vi "calc 3-phase ESR.vi"(7 "Acquisition mode":T1, 8 "error in":errorcluster, 10 "InverterWaveforms":T9, 11 "Processing loop variables":T2 {"CurrInverter"."last updated" format="%<%H:%M\n%d/%m/%Y>T"; "CurrInverter"."set flag" items=["False", "True"]}) -> (0 "error out":errorcluster, 1 "Max ESR":dbl[](array[numeric]), 2 "Raw ESR sum":dbl[](array[numeric]), 3 "Processing loop variables":T2 {"CurrInverter"."last updated" format="%<%H:%M\n%d/%m/%Y>T"; "CurrInverter"."set flag" items=["False", "True"]})   [LabVIEW 2019, in "Main.lvclass"]
doc: "Developed by Kevin Thompson\nkevin@thompsonengineering.net\n\nCopyright 2020\nThompson Engineering, LLC"
uses:
  Main.lvclass
  Common/DataTypes/InverterWaveforms--cluster.ctl
  Common/DataTypes/ChannelWaveforms--cluster.ctl
  DataTypes/Processing loop variables--cluster.ctl
  DataTypes/averaging variables.ctl
  DataTypes/ESR alarm variables.ctl
  Common/DataTypes/Inverter database record v2--cluster.ctl
  Common/DataTypes/inverter info v2--cluster.ctl
  Common/DataTypes/inverter gain range--cluster.ctl
  Common/DataTypes/inverter offset range--cluster.ctl
  Common/DataTypes/Acquisition Mode--cluster.ctl
  <vilib>/Analysis/baseanly.llb/Mean (DBL).vi
  <vilib>/Analysis/NI_AALPro.lvlib
  <vilib>/Analysis/NI_AALBase.lvlib
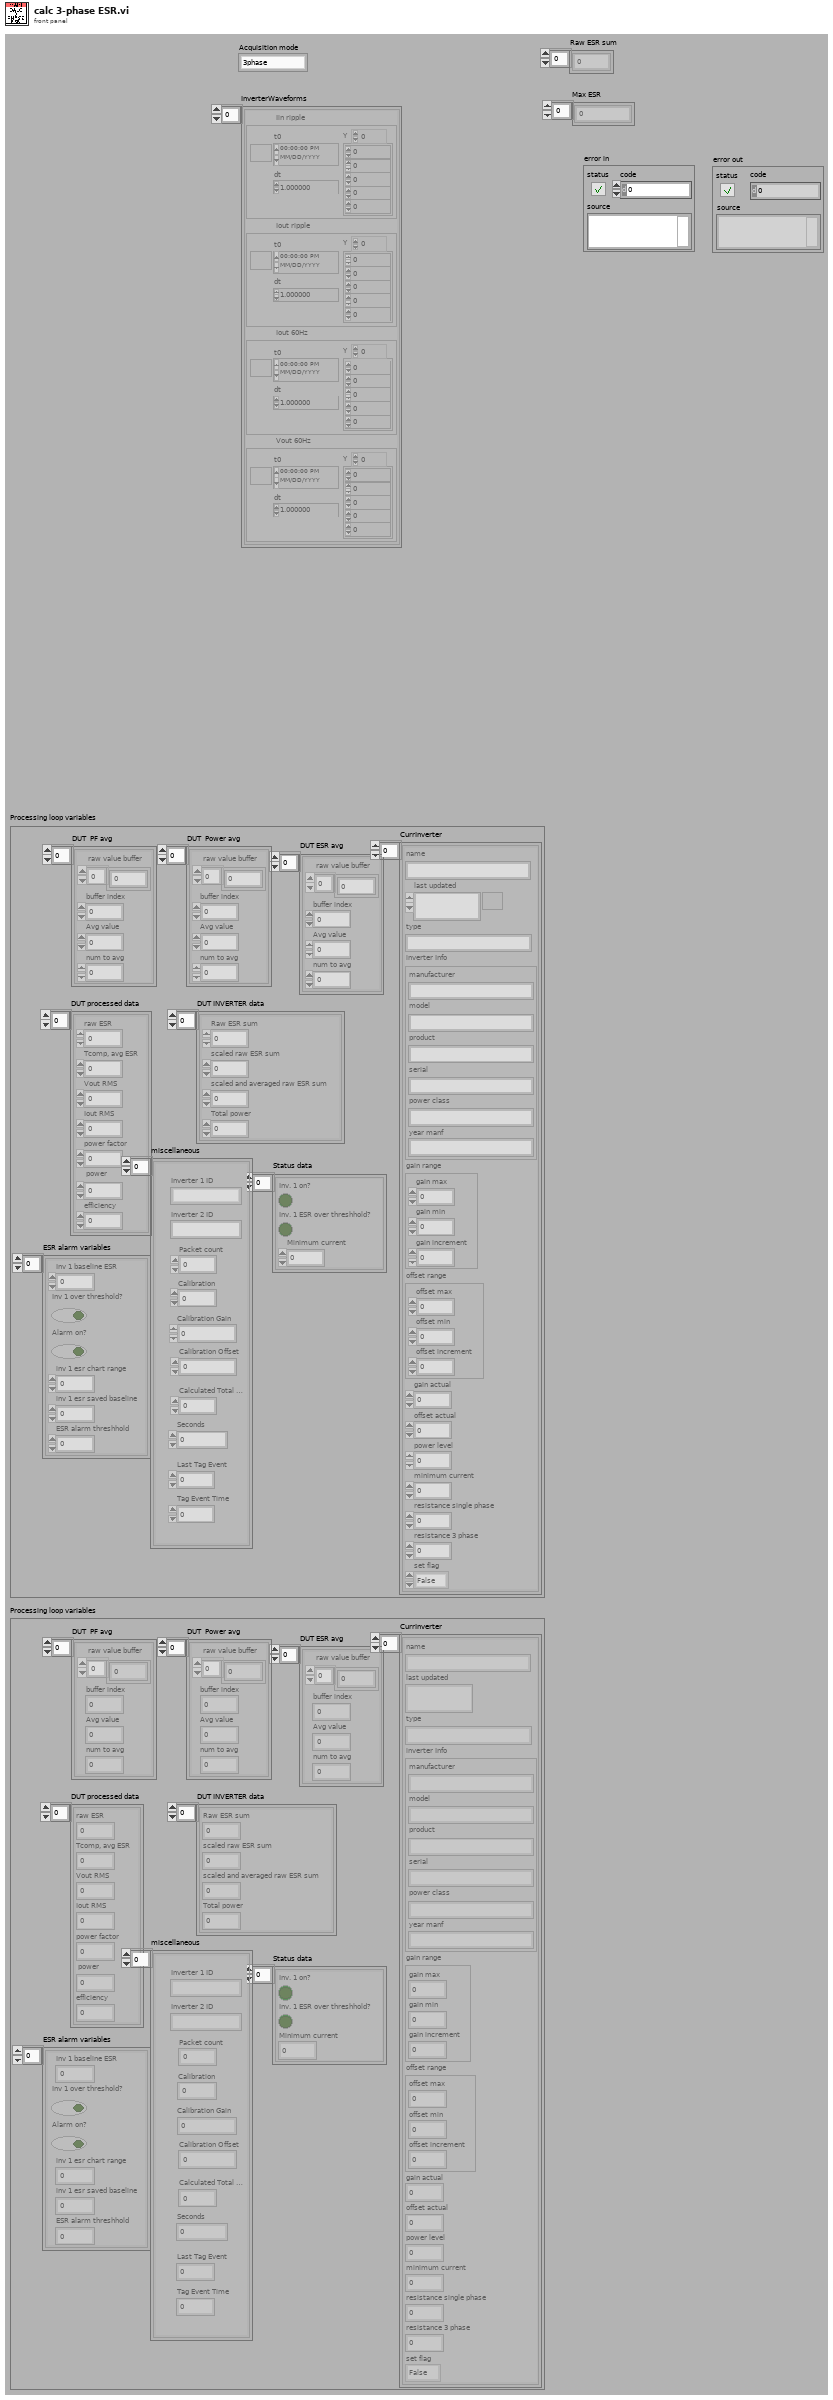
[diagram p1: front panel]
types:
  T1 = typedef "Acquisition Mode--cluster.ctl" = enum16{"3phase", "Single"}
  T2 = typedef "Main.lvclass/Processing loop variables--cluster.ctl" = cluster{"DUT ESR avg":T3[], "DUT  PF avg":T3[], "DUT  Power avg ":T3[], "DUT processed data":cluster{"raw ESR":dbl, "Tcomp, avg ESR":dbl, "Vout RMS":dbl, "Iout RMS":dbl, "power factor":dbl, "power":dbl, "efficiency":dbl}[], "ESR alarm variables":T4[], "Status data":cluster{"Inv. 1 on?":bool, "Inv. 1 ESR over threshhold?":bool, "Minimum current":dbl}[], "CurrInverter":T5[], "miscellaneous":cluster{"Inverter 1 ID":string, "Inverter 2 ID":string, "Packet count":u32, "Calibration":dbl, "Calibration Gain":dbl, "Calibration Offset":dbl, "Calculated Total Power":dbl, "Seconds":dbl, "Last Tag Event":dbl, "Tag Event Time":dbl}[], "DUT INVERTER data":cluster{"Raw ESR sum":dbl, "scaled raw ESR sum":dbl, "scaled and averaged raw ESR sum":dbl, "Total power":dbl}[]}
  T3 = typedef "Main.lvclass/averaging variables.ctl" = cluster{"raw value buffer":dbl[], "buffer index":i32, "Avg value":dbl, "num to avg":i32}
  T4 = typedef "Main.lvclass/ESR alarm variables.ctl" = cluster{"Inv 1 baseline ESR":dbl, "Inv 1 over threshold?":bool, "Alarm on?":bool, "inv 1 esr chart range":dbl, "inv 1 esr saved baseline":dbl, "ESR alarm threshhold":dbl}
  T5 = typedef "Inverter database record v2--cluster.ctl" = cluster{"name":string, "last updated":timestamp, "type":string, "inverter Info":T6, "gain range":T7, "offset range":T8, "gain actual":dbl, "offset actual":dbl, "power level":dbl, "minimum current":dbl, "resistance single phase":dbl, "resistance 3 phase":dbl, "set flag":u16}
  T6 = typedef "inverter info v2--cluster.ctl" = cluster{"manufacturer":string, "model":string, "product":string, "serial":string, "power class":string, "year manf":string}
  T7 = typedef "inverter gain range--cluster.ctl" = cluster{"gain max":dbl, "gain min":dbl, "gain increment":dbl}
  T8 = typedef "inverter offset range--cluster.ctl" = cluster{"offset max":dbl, "offset min":dbl, "offset increment":dbl}
  T9 = typedef "InverterWaveforms--cluster.ctl" = T10[]
  T10 = typedef "ChannelWaveforms--cluster.ctl" = cluster{"Iin ripple ":waveform(dbl), "Iout ripple ":waveform(dbl), "Iout 60Hz":waveform(dbl), "Vout 60Hz":waveform(dbl)}
  T11 = cluster{"raw ESR":dbl, "Tcomp, avg ESR":dbl, "Vout RMS":dbl, "Iout RMS":dbl, "power factor":dbl, "power":dbl, "efficiency":dbl}[]
  T12 = cluster{"Raw ESR sum":dbl, "scaled raw ESR sum":dbl, "scaled and averaged raw ESR sum":dbl, "Total power":dbl}[]
  T13 = cluster{"Raw ESR sum":dbl, "scaled raw ESR sum":dbl, "scaled and averaged raw ESR sum":dbl, "Total power":dbl}
  T14 = cluster{"raw ESR":dbl, "Tcomp, avg ESR":dbl, "Vout RMS":dbl, "Iout RMS":dbl, "power factor":dbl, "power":dbl, "efficiency":dbl}
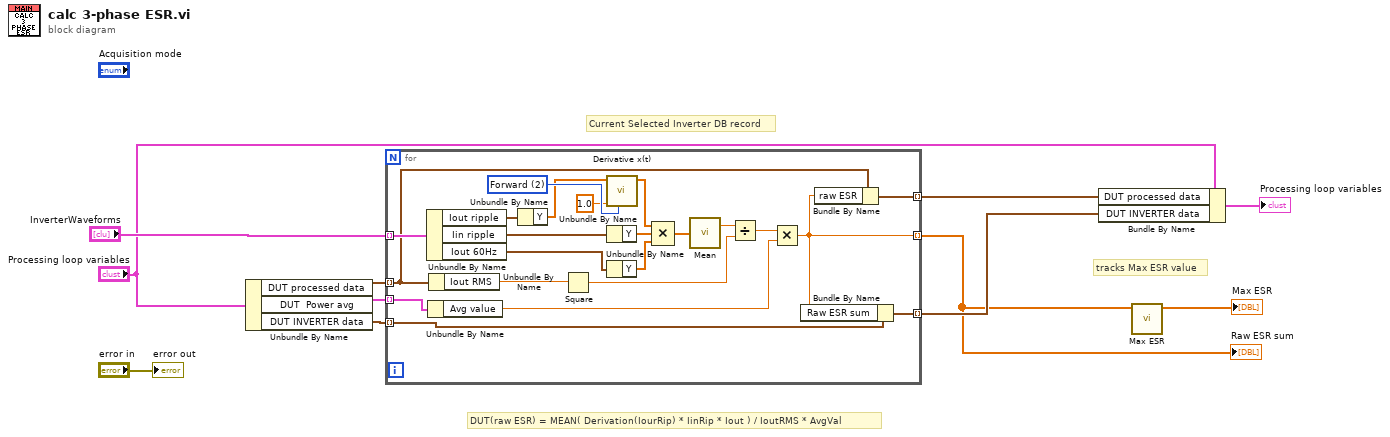
[diagram p0: block diagram]
diagram:
  # "DUT(raw ESR) = MEAN( Derivation(IourRip) * IinRip * Iout ) / IoutRMS * AvgVal"
  # "Current Selected Inverter DB record"
  # "tracks Max ESR value"
  n1 = Unbundle By Name("Processing loop variables") -> ("DUT processed data"=w8:T11, "DUT  Power avg"=w4:T3[], "DUT INVERTER data"=w3:T12)
  n2 = for {
    tunnel: "InverterWaveforms" -> [w23] mode=indexing
    tunnel: w8 -> [w16] mode=indexing
    tunnel: w4 -> [w19] mode=indexing
    tunnel: [w15] -> w6 mode=indexing
    tunnel: [w13] -> w1 mode=indexing
    tunnel: w3 -> [w14] mode=indexing
    tunnel: [w12] -> w2 mode=indexing
    w33 = u16 2 items=["2nd Order Central", "4th Order Central", "Forward", "Backward"] ("method")
    n3 = Unbundle By Name(w23) -> ("Iout ripple"=w22:waveform(dbl), "Iin ripple"=w21:waveform(dbl), "Iout 60Hz"=w20:waveform(dbl))
    n4 = Unbundle By Name(w19) -> ("Avg value"=w18:dbl)
    n5 = Unbundle By Name(w16) -> ("Iout RMS"=w17:dbl)
    n6 = Unbundle By Name(w22) -> ("Y"=w29:dbl[])
    n7 = Square(x=w17) -> (x^2=w30:dbl)
    n8 = call <vilib>:"Derivative x(t).vi"("method"=w33, "dt"=1.0, "X"=w29) -> ("dX/dt"=w27:dbl[])  [unwired: 7 in, 1 out]
    n9 = Unbundle By Name(w21) -> ("Y"=w26:dbl[])
    n10 = Unbundle By Name(w20) -> ("Y"=w25:dbl[])
    n11 = Compound Arithmetic op=MULTIPLY(w27, w26, w25) -> (w24:dbl[])
    n12 = call-poly <vilib>:"Mean.vi"("X"=w24) -> ("mean"=w28:dbl)  [unwired: 1 out]
    n13 = Divide(x=w28, y=w30) -> (x/y=w32:dbl)
    n14 = Multiply(x=w32, y=w18) -> (x*y=w13:dbl)
    n15 = Bundle By Name(cluster=w14, "Raw ESR sum"=w13) -> (w12:T13)
    n16 = Bundle By Name(cluster=w16, "raw ESR"=w13) -> (w15:T14)
  }
  "Raw ESR sum" <- w1
  n17 = Bundle By Name(cluster="Processing loop variables", "DUT processed data"=w6, "DUT INVERTER data"=w2) -> (→"Processing loop variables":T2)
  n18 = call "Max ESR.vi"("Raw ESR sum"=w1) -> ("Max ESR"=→"Max ESR":dbl[])  [unwired: 10 in]
  "error out" <- "error in"
